vi "U8_To_U32.vi"(0 "U32 IN":u32, 7 "U8 IN":u8) -> (4 "U8 OUT":u8, 8 "U32 OUT":u32)   [LabVIEW 2014]
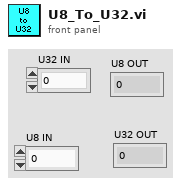
[diagram p1: front panel]
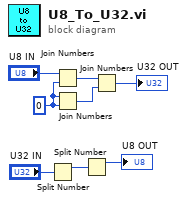
[diagram p0: block diagram]
diagram:
  w8 = u8 0
  n1 = Split Number(x="U32 IN") -> (hi(x)=w2:u16)  [unwired: 1 out]
  n2 = Join Numbers(hi="U8 IN", lo=w8) -> ((hi.lo)=w6:u16)
  n3 = Join Numbers(hi=w8, lo=w8) -> ((hi.lo)=w7:u16)
  n4 = Split Number(x=w2) -> (hi(x)=→"U8 OUT":u8)  [unwired: 1 out]
  n5 = Join Numbers(hi=w6, lo=w7) -> ((hi.lo)=→"U32 OUT":u32)
